vi "Exercise 3.1 – Manual Analysis.vi"() -> ()   [LabVIEW 2024]
panel:
  out "Frequency":dbl
  out "Amplitude":dbl
  in  "Frequency In":dbl(knob)=20.373516313769578 scale=0.0..100.0
  out "Waveform Graph":dynamicdata(graph)
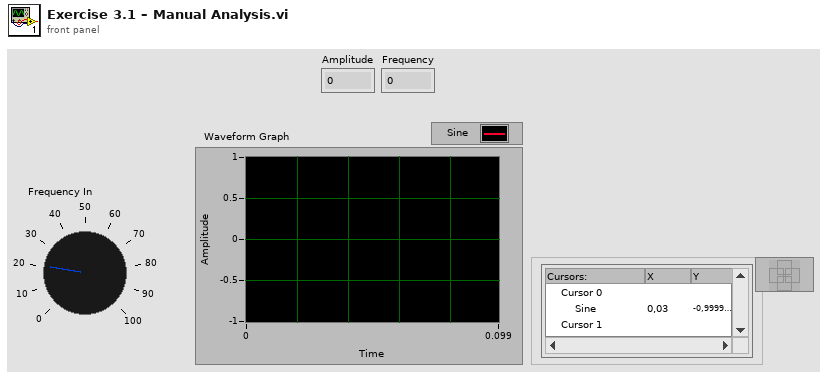
[diagram p1: front panel]
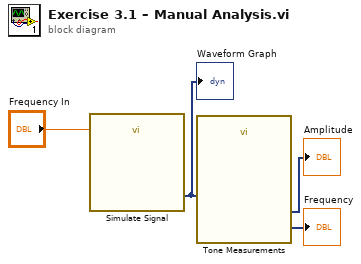
[diagram p0: block diagram]
diagram:
  n1 = call "Simulate Signal"("Frequency"="Frequency In") -> ("Sine"=w4:dynamicdata)  [unwired: 13 in, 1 out]
  "Waveform Graph" <- w4
  n2 = call "Tone Measurements"("Signals"=w4) -> ("Frequency"=→"Frequency":dynamicdata, "Amplitude"=→"Amplitude":dynamicdata)  [unwired: 8 in, 1 out]
